vi "多IP测试.vi"() -> ()   [LabVIEW 2019]
uses:
  <vilib>/Utility/miscctls.llb/LVPointTypeDef.ctl
panel:
  out "本机IP":string
  out "16记录":string[][](table)
  out "06记录":string[][](table)
  out "03记录（去重）":string[][](table)
  in  "选项卡控件":T1(tab)
  in  "簇 1":T2 caption="寄存器模拟"
  in  "簇 2":T2 caption="寄存器模拟"
  in  "簇 3":T2 caption="寄存器模拟"
  in  "簇 4":T2 caption="寄存器模拟"
  in  "簇 5":T2 caption="寄存器模拟"
  in  "簇 6":T2 caption="寄存器模拟"
  in  "簇 7":T2 caption="寄存器模拟"
  in  "簇 8":T2 caption="寄存器模拟"
  in  "簇 9":T2 caption="寄存器模拟"
  in  "初始化数组":bool
  in  "复位":bool
  in  "停止":bool
  in  "服务端地址":string="127.0.0.1"
  in  "远程端口":u16=4001
  in  "本地设置":T3={"0"={"连接设置"=FALSE, "本地端口"=5001}, "1"={"连接设置"=FALSE, "本地端口"=5002}, "2"={"连接设置"=FALSE, "本地端口"=5003}, "3"={"连接设置"=FALSE, "本地端口"=5004}, "4"={"连接设置"=FALSE, "本地端口"=5005}, "5"={"连接设置"=FALSE, "本地端口"=5006}, "6"={"连接设置"=FALSE, "本地端口"=5007}, "7"={"连接设置"=FALSE, "本地端口"=5008}, "8"={"连接设置"=FALSE, "本地端口"=5009}}
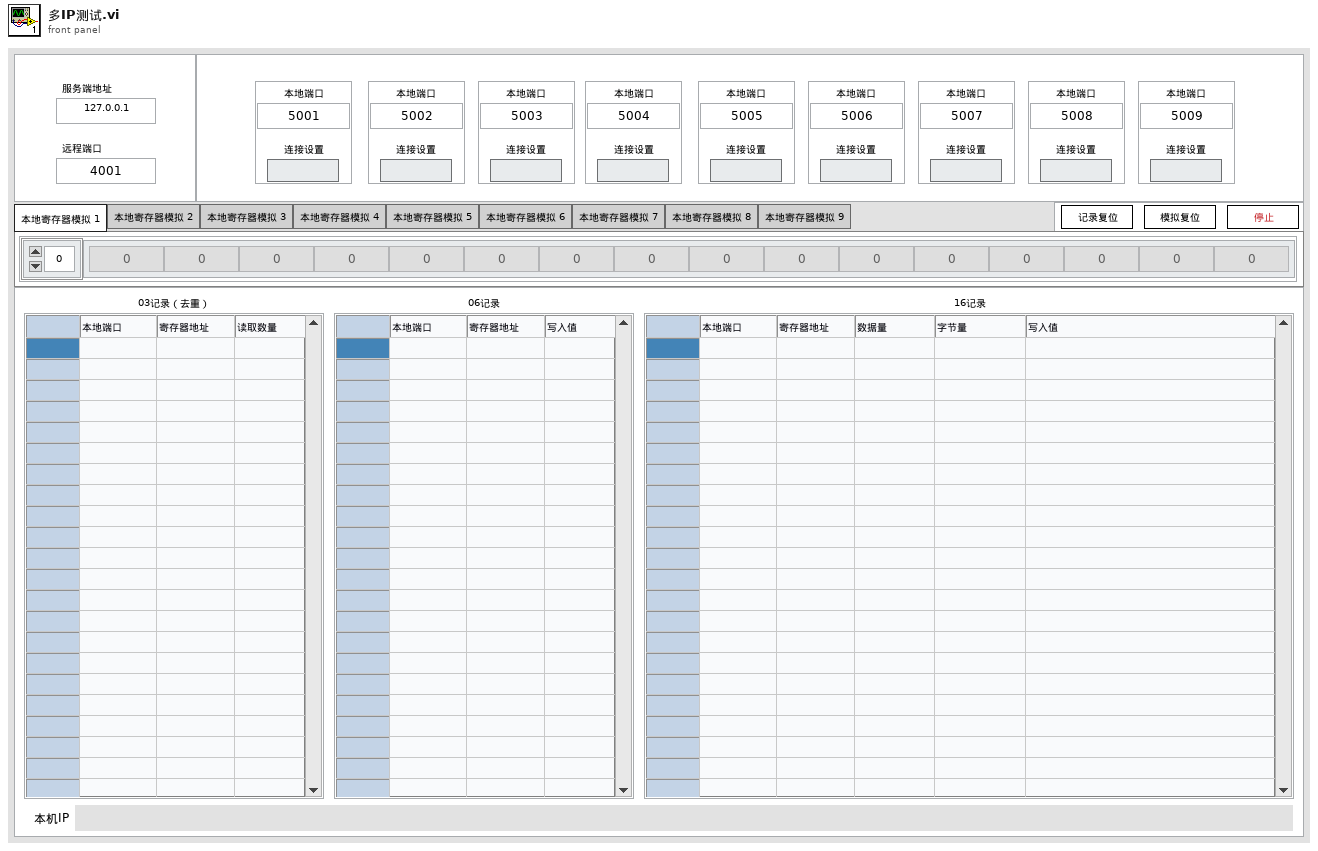
[diagram p1: front panel]
types:
  T1 = enum32{"本地寄存器模拟 1", "本地寄存器模拟 2", "本地寄存器模拟 3", "本地寄存器模拟 4", "本地寄存器模拟 5", "本地寄存器模拟 6", "本地寄存器模拟 7", "本地寄存器模拟 8", "本地寄存器模拟 9"}
  T2 = cluster{"03记录":string[][], "06记录":string[][], "16记录":string[][], "模拟数组":u16[]}
  T3 = cluster{"0":cluster{"连接设置":bool, "本地端口":u16}, "1":cluster{"连接设置":bool, "本地端口":u16}, "2":cluster{"连接设置":bool, "本地端口":u16}, "3":cluster{"连接设置":bool, "本地端口":u16}, "4":cluster{"连接设置":bool, "本地端口":u16}, "5":cluster{"连接设置":bool, "本地端口":u16}, "6":cluster{"连接设置":bool, "本地端口":u16}, "7":cluster{"连接设置":bool, "本地端口":u16}, "8":cluster{"连接设置":bool, "本地端口":u16}}
  T4 = typedef "LVPointTypeDef.ctl" = cluster{"Horizontal":i16, "Vertical":i16}
  T5 = cluster{"Label.Text":string, "NewVal":cluster{"连接设置":bool, "本地端口":u16}}
  T6 = cluster{"本地端口":u16, "模拟数组":u16[], "03记录":string[][], "06记录":string[][], "16记录":string[][]}
  T7 = cluster{"03记录":string[][], "06记录":string[][], "16记录":string[][], "模拟数组":u16[]}[]
  T8 = cluster{"本地端口":u16, u16[], "03记录":string[][], "06记录":string[][], "16记录":string[][]}
  T9 = cluster{"[0]":cluster{"连接设置":bool, "本地端口":u16}, "[1]":cluster{"连接设置":bool, "本地端口":u16}, "[2]":cluster{"连接设置":bool, "本地端口":u16}, "[3]":cluster{"连接设置":bool, "本地端口":u16}, "[4]":cluster{"连接设置":bool, "本地端口":u16}, "[5]":cluster{"连接设置":bool, "本地端口":u16}, "[6]":cluster{"连接设置":bool, "本地端口":u16}, "[7]":cluster{"连接设置":bool, "本地端口":u16}, "[8]":cluster{"连接设置":bool, "本地端口":u16}}
  T10 = cluster{"Value[0]":cluster{"连接设置":bool, "本地端口":u16}, "Value[1]":cluster{"连接设置":bool, "本地端口":u16}, "Value[2]":cluster{"连接设置":bool, "本地端口":u16}, "Value[3]":cluster{"连接设置":bool, "本地端口":u16}, "Value[4]":cluster{"连接设置":bool, "本地端口":u16}, "Value[5]":cluster{"连接设置":bool, "本地端口":u16}, "Value[6]":cluster{"连接设置":bool, "本地端口":u16}, "Value[7]":cluster{"连接设置":bool, "本地端口":u16}, "Value[8]":cluster{"连接设置":bool, "本地端口":u16}}
  T11 = cluster{"本地端口":u16, "模拟数组":u16[], "03记录":string[][], "06记录":string[][], "16记录":string[][]}[]
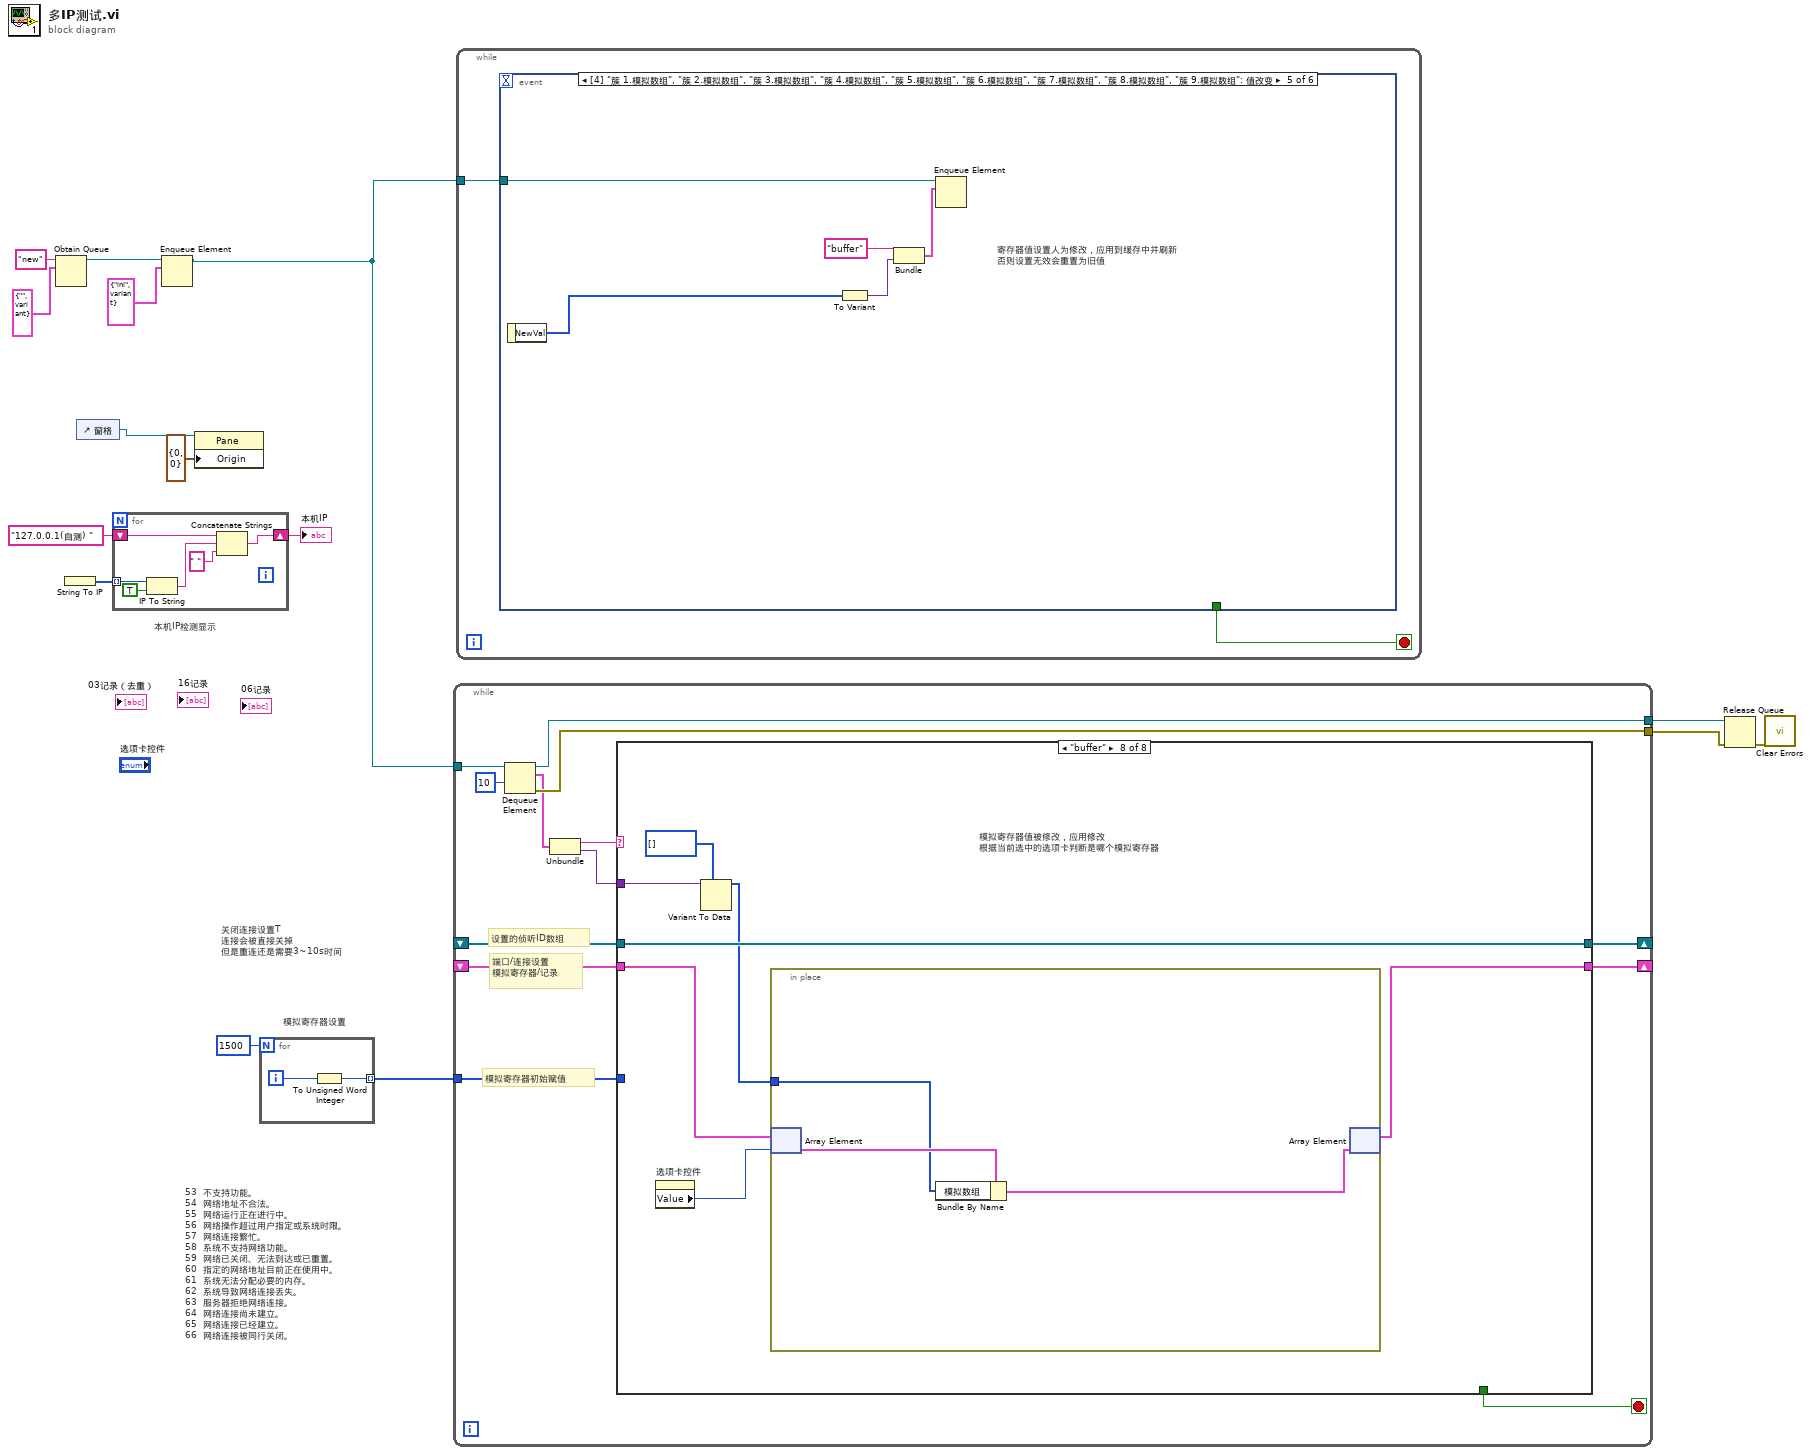
[diagram p0: block diagram]
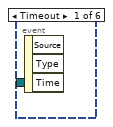
[diagram p2: hidden frame]
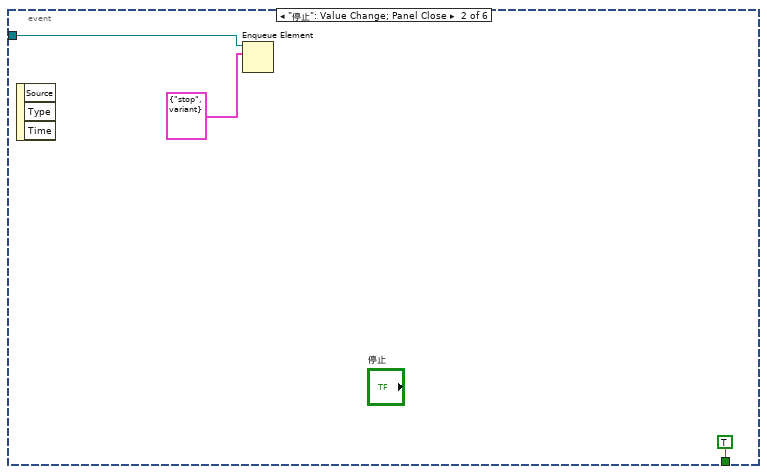
[diagram p3: hidden frame]
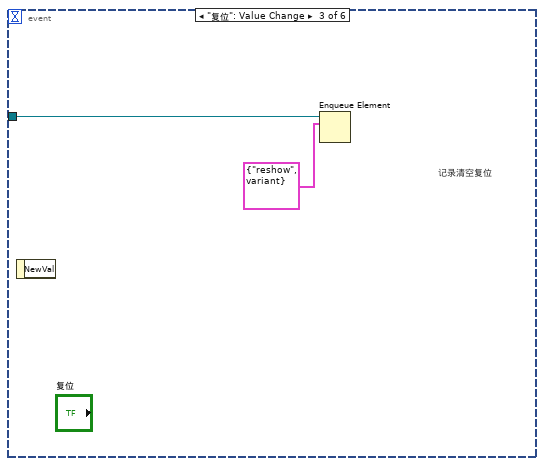
[diagram p4: hidden frame]
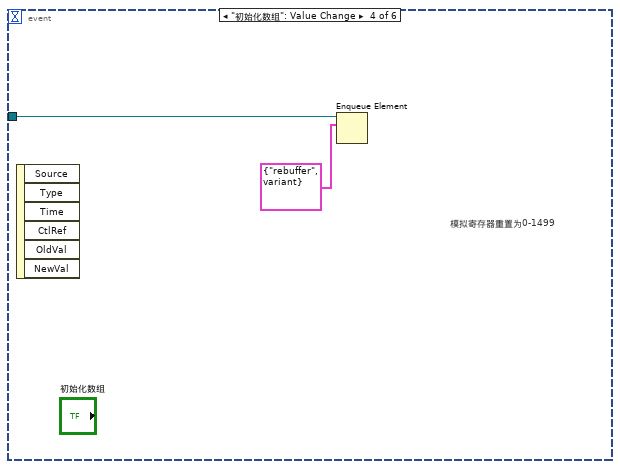
[diagram p5: hidden frame]
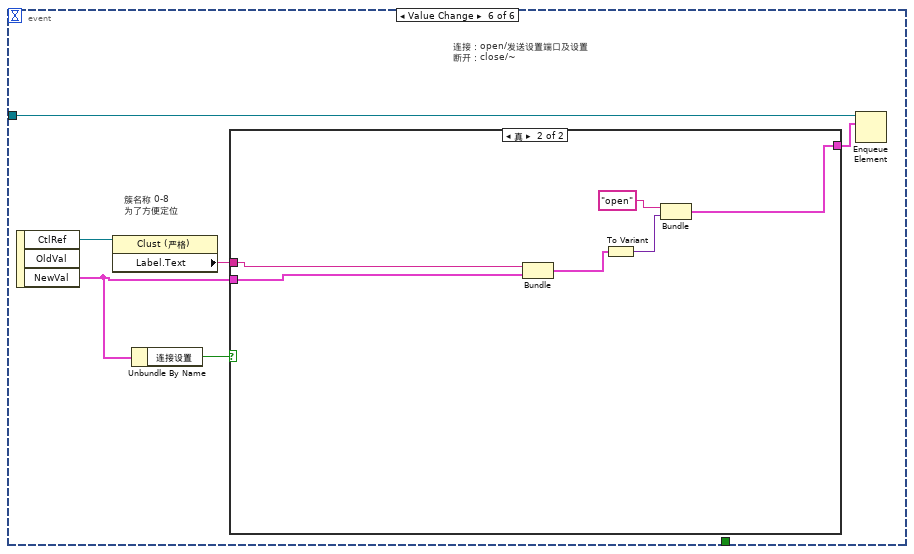
[diagram p6: hidden frame]
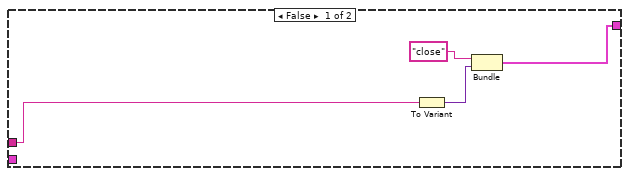
[diagram p7: hidden frame]
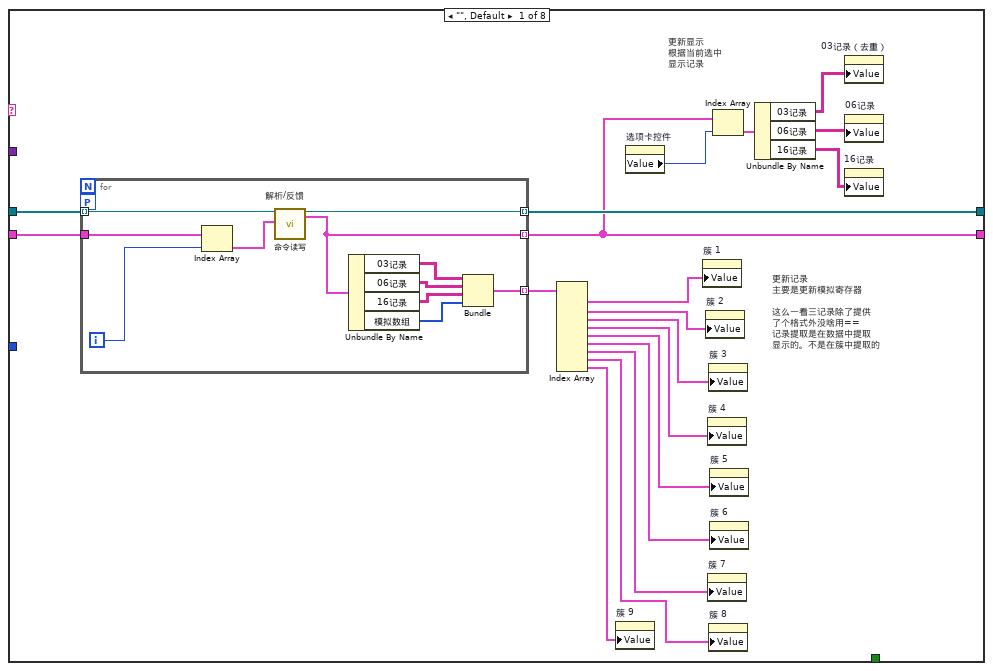
[diagram p8: hidden frame]
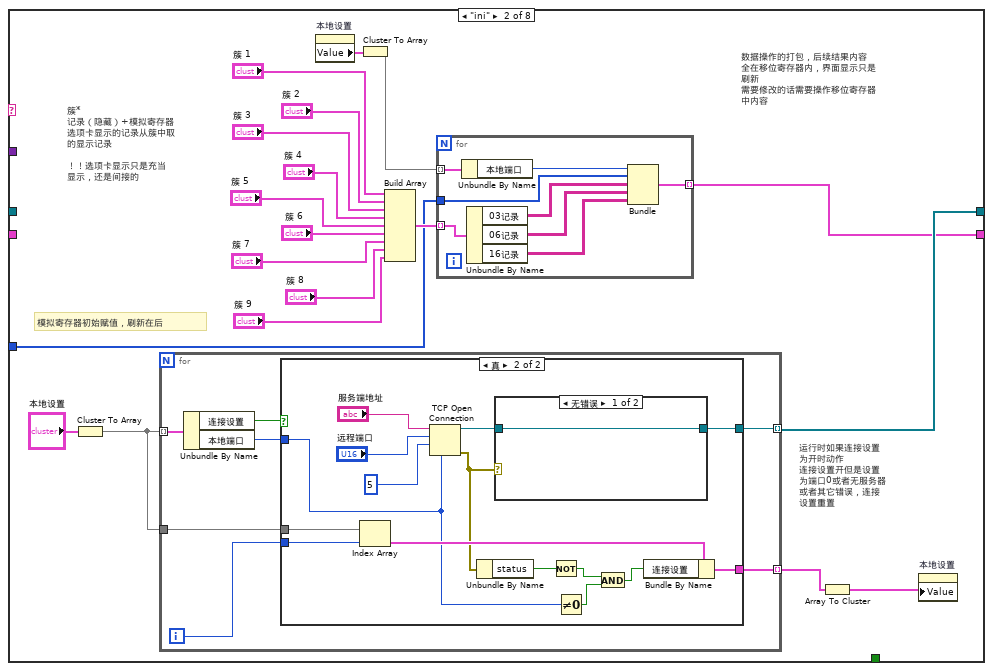
[diagram p9: hidden frame]
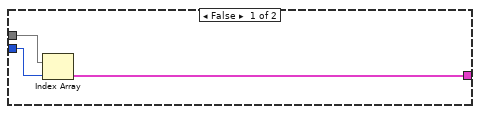
[diagram p10: hidden frame]
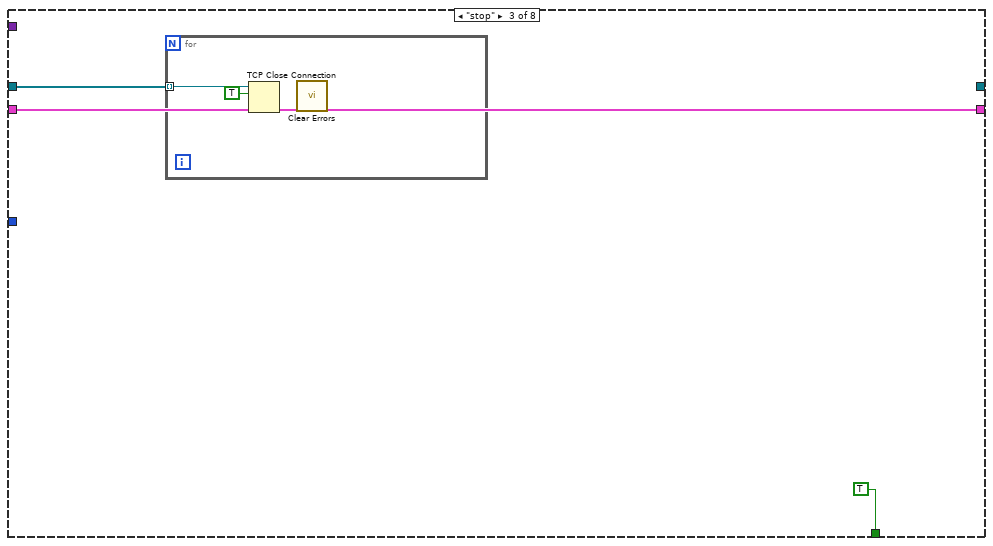
[diagram p12: hidden frame]
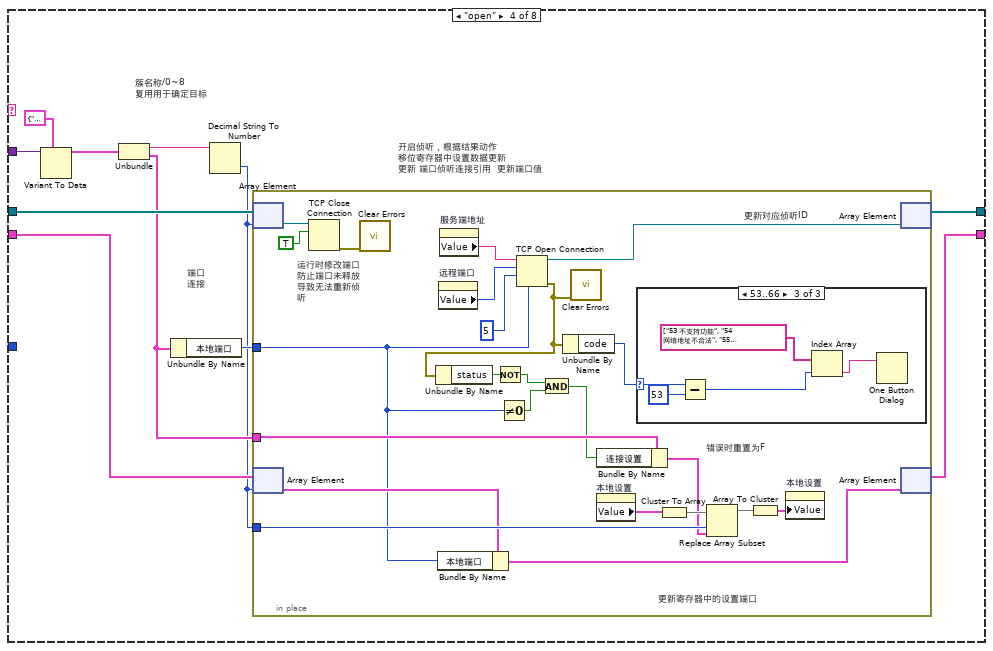
[diagram p13: hidden frame]
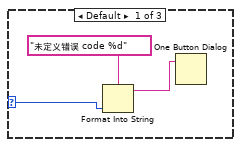
[diagram p14: hidden frame]
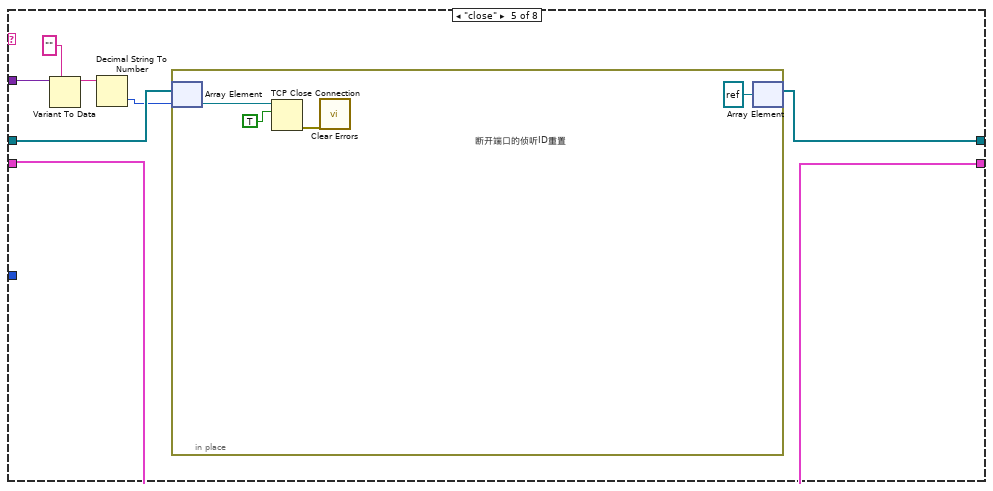
[diagram p16: hidden frame]
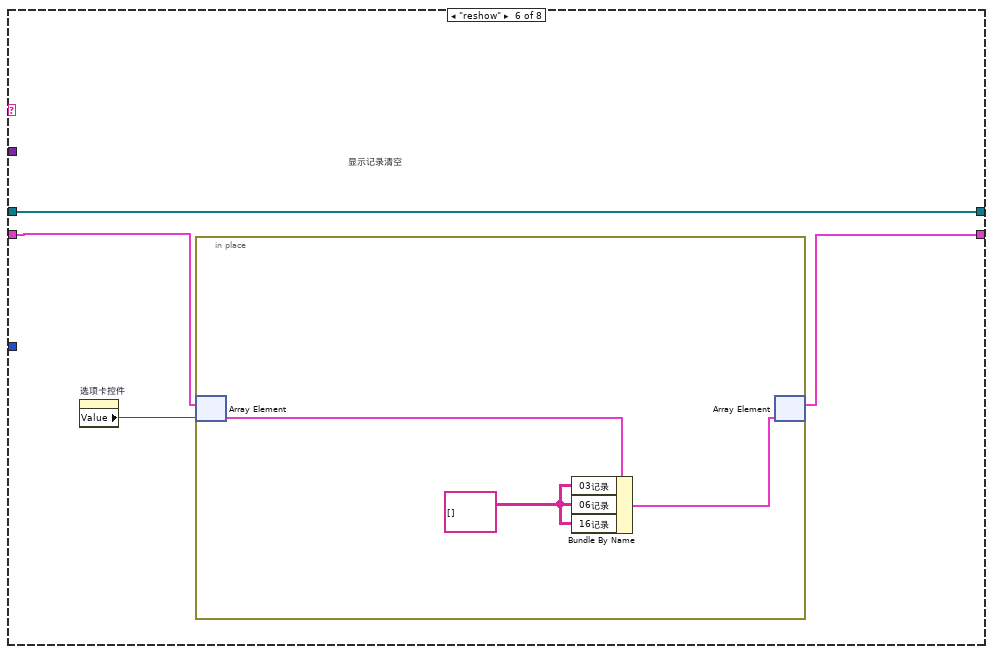
[diagram p17: hidden frame]
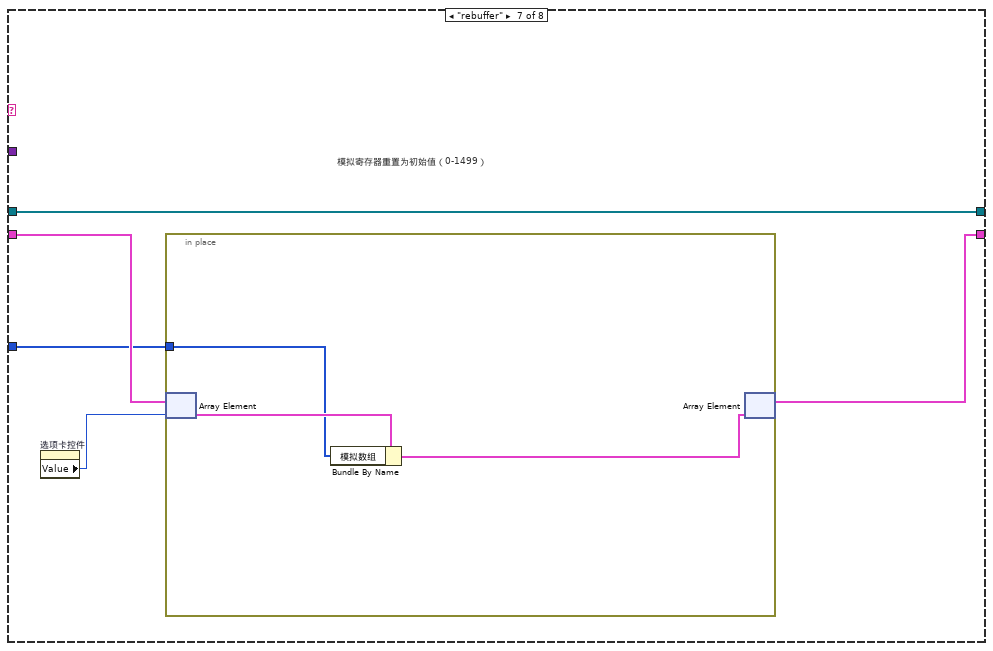
[diagram p18: hidden frame]
diagram:
  # "关闭连接设置T\n连接会被直接关掉\n但是重连还是需要3~10s时间"
  # "53  不支持功能。\n54  网络地址不合法。\n55  网络运行正在进行中。\n56  网络操作超过用户指定或系统时限。\n57  网络连接繁忙。\n58  系统不支持网络功能。\n59  网络已关闭、无法到达或已重置。\n60  指定的网络地址目前正在使用中。\n61  系统无法分配必要的内存。\n62  系统导致网络连接丢失。\n63  服务器拒绝网络连接。\n64  网络连接尚未建立。\n65  网络连接已经建立。\n66  网络连接被同行关闭。"
  # "本机IP检测显示"
  # "模拟寄存器设置"
  n1 = Obtain Queue(name (unnamed)="new" ("名称（未命名）"), element data type=cluster{"元素":string, variant} {"元素"="", variant}) -> (queue out=w14:refnum<queue>)  [unwired: 3 in, 2 out]
  n2 = String To IP() -> (0:w2:u32[])  [unwired: 1 in]
  n3 = control-ref of="窗格"() -> (w7:refnum<vi>)
  n4 = for {
    tunnel: w2 -> [w21] mode=indexing
    shift-right: [w18] -> w3
    shift-left: "127.0.0.1(自测) " ("name") -> [w19]
    n5 = IP To String(1:TRUE ("句点符号？(F)"), 2:w21) -> (0:w17:string)
    n6 = Concatenate Strings(w19, w17, " " ("字符串")) -> (w18:string)
  }
  "本机IP" <- w3
  n7 = Enqueue Element(queue=w14, element=cluster{"元素":string, variant} {"元素"="ini", variant}) -> (queue out=w8:refnum<queue>)  [unwired: 2 in, 2 out]
  n8 = property class="Pane"(reference=w7, "Origin"=T4 {"Horizontal"=0, "Vertical"=0} ("原点")) -> ()  [unwired: 1 in, 2 out]
  n9 = for {
    N: 1500 -> [_]
    tunnel: [w22] -> w4 mode=indexing
    i -> [w23]
    n10 = To Unsigned Word Integer(number=w23) -> (unsigned 16bit integer=w22:u16)
  }
  n11 = while {
    tunnel: w8 -> [w36]
    shift-right: [w35] -> _
    shift-left: _ -> [w30]
    tunnel: [w33] -> w12
    tunnel: [w32] -> w11
    shift-right: [w25] -> _
    shift-left: _ -> [w26]
    tunnel: w4 -> [w24]
    stop <- w34 stop-if-true
    # "设置的侦听ID数组"
    # "端口/连接设置\n模拟寄存器/记录"
    # "模拟寄存器初始赋值"
    n12 = Dequeue Element(queue=w36, timeout in ms (-1)=10 ("超时毫秒(-1)")) -> (queue out=w33:refnum<queue>, element=w29:cluster{"元素":string, variant}, error out=w32:errorcluster)  [unwired: 1 in, 1 out]
    n13 = Unbundle(w29) -> ("元素"=w28:string, w27:variant)
    n14 = case shown="\"buffer\"" w28 {
      tunnel: [w54 w84 _ w134 w172 w183 w191 w201] -> w35
      tunnel: [_ _ TRUE _ _ _ _ _] -> w34
      tunnel: w30 -> [w55 _ w121 w135 w171 w183 w191 w201]
      tunnel: w27 -> [_ _ _ w137 w174 _ _ w200]
      tunnel: w26 -> [w53 _ w122 w128 w169 w181 w189 w198]
      tunnel: [w52 w68 w122 w129 w169 w180 w188 w197] -> w25
      tunnel: w24 -> [_ w67 _ _ _ _ w187 _]
      frame "", Default {
        # "更新显示\n根据当前选中\n显示记录"
        # "更新记录\n主要是更新模拟寄存器\n\n这么一看三记录除了提供\n了个格式外没啥用==\n记录提取是在数据中提取\n显示的。不是在簇中提取的"
        n15 = for {
          tunnel: w55 -> [w66] mode=indexing
          tunnel: [w65] -> w54 mode=indexing
          tunnel: w53 -> [w63]
          tunnel: [w61] -> w52 mode=indexing
          tunnel: [w56] -> w46 mode=indexing
          workers-P: _ -> [_]
          i -> [w64]
          # "解析/反馈"
          n16 = Index Array(array=w63, index=w64) -> (element=w62:T6)
          n17 = call "命令读写.vi"("连接ID"=w66, "输入簇"=w62) -> ("连接ID输出"=w65:refnum<k5>, "输出簇"=w61:T6)  [unwired: 16 in]
          n18 = Unbundle By Name(w61) -> ("03记录"=w60:string[][], "06记录"=w59:string[][], "16记录"=w58:string[][], "模拟数组"=w57:u16[])
          n19 = Bundle("03记录"=w60, "06记录"=w59, "16记录"=w58, "模拟数组"=w57) -> (w56:T2)  [unwired: 1 in]
        }
        n20 = Index Array(array=w46) -> (element #1=w45:T2, element #2=w44:T2, element #3=w43:T2, element #4=w40:T2, element #5=w39:T2, element #6=w38:T2, element #7=w37:T2, element #8=w41:T2, element #9=w42:T2)  [unwired: 9 in]
        n21 = property on="簇 9" class="Clust (严格)"("Value"=w42) -> ()  [unwired: 2 in, 2 out]
        n22 = property on="选项卡控件" class="TabCtl (严格)"() -> ("Value"=w51:T1)  [unwired: 2 in, 2 out]
        n23 = property on="簇 1" class="Clust (严格)"("Value"=w45) -> ()  [unwired: 2 in, 2 out]
        n24 = property on="簇 2" class="Clust (严格)"("Value"=w44) -> ()  [unwired: 2 in, 2 out]
        n25 = property on="簇 4" class="Clust (严格)"("Value"=w40) -> ()  [unwired: 2 in, 2 out]
        n26 = property on="簇 7" class="Clust (严格)"("Value"=w37) -> ()  [unwired: 2 in, 2 out]
        n27 = property on="簇 3" class="Clust (严格)"("Value"=w43) -> ()  [unwired: 2 in, 2 out]
        n28 = property on="簇 8" class="Clust (严格)"("Value"=w41) -> ()  [unwired: 2 in, 2 out]
        n29 = property on="簇 5" class="Clust (严格)"("Value"=w39) -> ()  [unwired: 2 in, 2 out]
        n30 = property on="簇 6" class="Clust (严格)"("Value"=w38) -> ()  [unwired: 2 in, 2 out]
        n31 = Index Array(array=w52, index=w51) -> (element=w50:T6)
        n32 = Unbundle By Name(w50) -> ("03记录"=w47:string[][], "06记录"=w49:string[][], "16记录"=w48:string[][])
        n33 = property on="03记录（去重）" class="Tbl (严格)"("Value"=w47) -> ()  [unwired: 2 in, 2 out]
        n34 = property on="06记录" class="Tbl (严格)"("Value"=w49) -> ()  [unwired: 2 in, 2 out]
        n35 = property on="16记录" class="Tbl (严格)"("Value"=w48) -> ()  [unwired: 2 in, 2 out]
      }
      frame "ini" {
        # "数据操作的打包，后续结果内容\n全在移位寄存器内，界面显示只是\n刷新\n需要修改的话需要操作移位寄存器\n中内容"
        # "运行时如果连接设置\n为开时动作\n连接设置开但是设置\n为端口0或者无服务器\n或者其它错误，连接\n设置重置"
        # "模拟寄存器初始赋值，刷新在后"
        # "簇*\n记录（隐藏）+模拟寄存器\n选项卡显示的记录从簇中取\n的显示记录\n\n！！选项卡显示只是充当\n显示，还是间接的"
        n36 = Cluster To Array(cluster="本地设置") -> (array=w83:cluster{"连接设置":bool, "本地端口":u16}[])
        n37 = for {
          tunnel: w83 -> [w100] mode=indexing
          tunnel: [w97] -> w84 mode=indexing
          tunnel: w83 -> [w96]
          tunnel: [w94] -> w81 mode=indexing
          i -> [w95]
          n38 = Unbundle By Name(w100) -> ("连接设置"=w99:bool, "本地端口"=w98:u16)
          n39 = case shown="真" w99 {
            tunnel: w98 -> [_ w107]
            tunnel: [_ w115] -> w97
            tunnel: w96 -> [w102 w113]
            tunnel: w95 -> [w103 w112]
            tunnel: [w101 w109] -> w94
            frame False {
              n40 = Index Array(array=w102, index=w103) -> (element=w101:cluster{"连接设置":bool, "本地端口":u16})
            }
            frame True {
              n41 = Index Array(array=w113, index=w112) -> (element=w111:cluster{"连接设置":bool, "本地端口":u16})
              n42 = TCP Open Connection(address="服务端地址", remote port or service name="远程端口", timeout ms (60000)=5 ("超时毫秒(60000)"), local port=w107) -> (connection ID=w114:refnum<k5>, error out=w110:errorcluster)  [unwired: 1 in]
              n43 = Unbundle By Name(w110) -> ("status"=w108:bool)
              n44 = case shown="无错误" w110 {
                tunnel: [w119 w120] -> w115
                tunnel: w114 -> [w119 w120]
                frame No Error {
                }
                frame Default {
                }
              }
              n45 = Not(x=w108) -> (.not. x?=w106:bool)
              n46 = Not Equal To 0?(x=w107) -> (x != 0?=w105:bool)
              n47 = And(x=w106, y=w105) -> (x .and. y?=w104:bool)
              n48 = Bundle By Name(cluster=w111, "连接设置"=w104) -> (w109:cluster{"连接设置":bool, "本地端口":u16})
            }
          }
        }
        n49 = property on="本地设置" class="Clust (严格)"() -> ("Value"=w78:T3)  [unwired: 2 in, 2 out]
        n50 = Cluster To Array(cluster=w78) -> (array=w79:cluster{"连接设置":bool, "本地端口":u16}[])
        n51 = Build Array("簇 1", "簇 2", "簇 3", "簇 4", "簇 5", "簇 6", "簇 7", "簇 8", "簇 9") -> (w80:T7)
        n52 = for {
          tunnel: w79 -> [w93] mode=indexing
          tunnel: w80 -> [w90] mode=indexing
          tunnel: [w92] -> w68 mode=indexing
          tunnel: w67 -> [w86]
          n53 = Unbundle By Name(w93) -> ("本地端口"=w91:u16)
          n54 = Unbundle By Name(w90) -> ("03记录"=w89:string[][], "06记录"=w88:string[][], "16记录"=w87:string[][])
          n55 = Bundle("本地端口"=w91, w86, "03记录"=w89, "06记录"=w88, "16记录"=w87) -> (w92:T8)  [unwired: 1 in]
        }
        n56 = Array To Cluster(array=w81) -> (cluster=w82:T9)
        n57 = property on="本地设置" class="Clust (严格)"("Value"=w82) -> ()  [unwired: 2 in, 2 out]
      }
      frame "stop" {
        n58 = for {
          tunnel: w121 -> [w125] mode=indexing
          n59 = TCP Close Connection(connection ID=w125, abort (F)=TRUE ("中止(F)")) -> (error out=w126:errorcluster)  [unwired: 1 in, 1 out]
          n60 = call <vilib>:"Clear Errors.vi"("error in (no error)"=w126) -> ()  [unwired: 5 in, 2 out]
        }
      }
      frame "open" {
        # "端口\n连接"
        # "簇名称/0~8\n复用用于确定目标"
        # "开启侦听，根据结果动作\n移位寄存器中设置数据更新\n更新 端口侦听连接引用  更新端口值"
        n61 = Variant To Data(type=T5 {"Label.Text"="", "NewVal"={"连接设置"=FALSE, "本地端口"=0}} ("输出簇"), Variant=w137) -> (data=w136:T5)  [unwired: 1 in, 1 out]
        n62 = Unbundle(w136) -> ("Label.Text"=w131:string, "NewVal"=w130:cluster{"连接设置":bool, "本地端口":u16})
        n63 = Unbundle By Name(w130) -> ("本地端口"=w133:u16)
        n64 = Decimal String To Number(string=w131) -> (number=w127:i32)  [unwired: 2 in, 1 out]
        n65 = in-place {
          in-place-border: w133 -> [w144]
          in-place-border: w127 -> [w151]
          in-place-border: w130 -> [w150]
          # "运行时修改端口\n防止端口未释放\n导致无法重新侦\n听"
          # "更新寄存器中的设置端口"
          # "更新对应侦听ID"
          # "错误时重置为F"
          n66 = in-place-array #1(w135, w127) -> (w142:refnum<k5>)
          n67 = in-place-array #2(w128, w127) -> (w145:T6)
          n68 = TCP Close Connection(connection ID=w142, abort (F)=TRUE ("中止(F)")) -> (error out=w141:errorcluster)  [unwired: 1 in, 1 out]
          n69 = call <vilib>:"Clear Errors.vi"("error in (no error)"=w141) -> ()  [unwired: 5 in, 2 out]
          n70 = Bundle By Name(cluster=w145, "本地端口"=w144) -> (w143:T6)
          n71 = property on="远程端口" class="DigNum (严格)"() -> ("Value"=w158:u16)  [unwired: 2 in, 2 out]
          n72 = property on="服务端地址" class="Str"() -> ("Value"=w159:string)  [unwired: 2 in, 2 out]
          n73 = Not Equal To 0?(x=w144) -> (x != 0?=w156:bool)
          n74 = TCP Open Connection(address=w159, remote port or service name=w158, timeout ms (60000)=5 ("超时毫秒(60000)"), local port=w144) -> (connection ID=w157:refnum<k5>, error out=w140:errorcluster)  [unwired: 1 in]
          n75 = Unbundle By Name(w140) -> ("status"=w154:bool)
          n76 = Not(x=w154) -> (.not. x?=w155:bool)
          n77 = And(x=w155, y=w156) -> (x .and. y?=w146:bool)
          n78 = Unbundle By Name(w140) -> ("code"=w139:i32)
          n79 = call <vilib>:"Clear Errors.vi"("error in (no error)"=w140) -> ()  [unwired: 5 in, 2 out]
          n80 = Bundle By Name(cluster=w150, "连接设置"=w146) -> (w149:cluster{"连接设置":bool, "本地端口":u16})
          n81 = property on="本地设置" class="Clust (严格)"() -> ("Value"=w152:T3)  [unwired: 2 in, 2 out]
          n82 = case shown="53..66" w139 {
            selector: w139 -> [w163 _ w168]
            frame Default {
              n83 = Format Into String(format string="未定义错误 code %d" ("格式字符串"), w163) -> (resulting string=w162:string)  [unwired: 2 in, 1 out]
              n84 = One Button Dialog(message=w162) -> ()  [unwired: 1 in, 1 out]
            }
            frame 0 {
            }
            frame 53..66 {
              n85 = Subtract(x=w168, y=53) -> (x-y=w165:i32)
              n86 = Index Array(array=string[] ["53 不支持功能", "54 网络地址不合法", "55 网络运行正在进行中", "56 网络操作超过用户指定或系统时限", "57 网络连接繁忙", "58 系统不支持网络功能", "59 网络已关闭、无法到达或已重置。", "60 指定的网络地址目前正在使用中", "61 系统无法分配必要的内存", "62 系统导致网络连接丢失", "63 服务器拒绝网络连接", "64 网络连接尚未建立", "65 网络连接已经建立", "66 网络连接被同行关闭"], index=w165) -> (element=w164:string)
              n87 = One Button Dialog(message=w164) -> ()  [unwired: 1 in, 1 out]
            }
          }
          n88 = Cluster To Array(cluster=w152) -> (array=w153:cluster{"连接设置":bool, "本地端口":u16}[])
          n89 = Replace Array Subset(array=w153, new element=w149, index=w151) -> (w148:cluster{"连接设置":bool, "本地端口":u16}[])
          n90 = Array To Cluster(array=w148) -> (cluster=w147:T10)
          n91 = property on="本地设置" class="Clust (严格)"("Value"=w147) -> ()  [unwired: 2 in, 2 out]
          n92 = in-place-array #1(w157) -> (w134:refnum<k5>[])  [unwired: 1 out]
          n93 = in-place-array #2(w143) -> (w129:T11)  [unwired: 1 out]
        }
      }
      frame "close" {
        n94 = Variant To Data(type="", Variant=w174) -> (data=w173:string)  [unwired: 1 in, 1 out]
        n95 = Decimal String To Number(string=w173) -> (number=w170:i32)  [unwired: 2 in, 1 out]
        n96 = in-place {
          # "断开端口的侦听ID重置"
          n97 = in-place-array #3(w171, w170) -> (w178:refnum<k5>)
          n98 = TCP Close Connection(connection ID=w178, abort (F)=TRUE ("中止(F)")) -> (error out=w177:errorcluster)  [unwired: 1 in, 1 out]
          n99 = call <vilib>:"Clear Errors.vi"("error in (no error)"=w177) -> ()  [unwired: 5 in, 2 out]
          n100 = in-place-array #3(refnum<k5> refnum ("元素")) -> (w172:refnum<k5>[])  [unwired: 1 out]
        }
      }
      frame "reshow" {
        # "显示记录清空"
        n101 = property on="选项卡控件" class="TabCtl (严格)"() -> ("Value"=w182:T1)  [unwired: 2 in, 2 out]
        n102 = in-place {
          w185 = string[][] [] ("03记录")
          n103 = in-place-array #4(w181, w182) -> (w184:T6)
          n104 = Bundle By Name(cluster=w184, "03记录"=w185, "06记录"=w185, "16记录"=w185) -> (w186:T6)
          n105 = in-place-array #4(w186) -> (w180:T11)  [unwired: 1 out]
        }
      }
      frame "rebuffer" {
        # "模拟寄存器重置为初始值（0-1499）"
        n106 = property on="选项卡控件" class="TabCtl (严格)"() -> ("Value"=w190:T1)  [unwired: 2 in, 2 out]
        n107 = in-place {
          in-place-border: w187 -> [w193]
          n108 = in-place-array #5(w189, w190) -> (w194:T6)
          n109 = Bundle By Name(cluster=w194, "模拟数组"=w193) -> (w192:T6)
          n110 = in-place-array #5(w192) -> (w188:T11)  [unwired: 1 out]
        }
      }
      frame "buffer" {
        # "模拟寄存器值被修改，应用修改\n根据当前选中的选项卡判断是哪个模拟寄存器"
        n111 = property on="选项卡控件" class="TabCtl (严格)"() -> ("Value"=w195:T1)  [unwired: 2 in, 2 out]
        n112 = Variant To Data(type=u16[] [] ("新值"), Variant=w200) -> (data=w196:u16[])  [unwired: 1 in, 1 out]
        n113 = in-place {
          in-place-border: w196 -> [w203]
          n114 = in-place-array #6(w198, w195) -> (w204:T6)
          n115 = Bundle By Name(cluster=w204, "模拟数组"=w203) -> (w202:T6)
          n116 = in-place-array #6(w202) -> (w197:T11)  [unwired: 1 out]
        }
      }
    }
  }
  n117 = while {
    tunnel: w8 -> [w206]
    stop <- w205 stop-if-true
    n118 = event shown="[4] \"簇 1.模拟数组\", \"簇 2.模拟数组\", \"簇 3.模拟数组\", \"簇 4.模拟数组\", \"簇 5.模拟数组\", \"簇 6.模拟数组\", \"簇 7.模拟数组\", \"簇 8.模拟数组\", \"簇 9.模拟数组\": 值改变" {
      selector: _ -> [_ _ _ _ _ _]
      dyn-events: _ -> [_ _ _ _ _ _]
      timeout: _ -> [_ _ _ _ _ _]
      tunnel: w206 -> [_ w209 w210 w212 w214 w224]
      tunnel: [_ TRUE ("停止") _ _ _ _] -> w205
      event Timeout {
        n119 = event-data() -> ()  [unwired: 1 in, 3 out]
      }
      event "停止": Value Change; Panel Close {
        n120 = event-data() -> ()  [unwired: 1 in, 3 out]
        n121 = Enqueue Element(queue=w209, element=cluster{"元素":string, variant} {"元素"="stop", variant}) -> ()  [unwired: 2 in, 3 out]
      }
      event "复位": Value Change {
        # "记录清空复位"
        n122 = event-data() -> ()  [unwired: 1 in, 1 out]
        n123 = Enqueue Element(queue=w210, element=cluster{"元素":string, variant} {"元素"="reshow", variant}) -> ()  [unwired: 2 in, 3 out]
      }
      event "初始化数组": Value Change {
        # "模拟寄存器重置为0-1499"
        n124 = event-data() -> ()  [unwired: 1 in, 6 out]
        n125 = Enqueue Element(queue=w212, element=cluster{"元素":string, variant} {"元素"="rebuffer", variant}) -> ()  [unwired: 2 in, 3 out]
      }
      event "簇 1.模拟数组", "簇 2.模拟数组", "簇 3.模拟数组", "簇 4.模拟数组", "簇 5.模拟数组", "簇 6.模拟数组", "簇 7.模拟数组", "簇 8.模拟数组", "簇 9.模拟数组": Value Change {
        # "寄存器值设置人为修改，应用到缓存中并刷新\n否则设置无效会重置为旧值"
        n126 = event-data() -> ("NewVal"=w218:u16[])  [unwired: 1 in]
        n127 = To Variant(anything=w218) -> (Variant=w216:variant)
        n128 = Bundle("元素"="buffer", "Variant"=w216) -> (w215:cluster{"元素":string, "Variant":variant})  [unwired: 1 in]
        n129 = Enqueue Element(queue=w214, element=w215) -> ()  [unwired: 2 in, 3 out]
      }
      event "本地设置.0", "本地设置.1", "本地设置.2", "本地设置.3", "本地设置.4", "本地设置.5", "本地设置.6", "本地设置.7", "本地设置.8": Value Change {
        # "簇名称 0-8\n为了方便定位"
        # "连接：open/发送设置端口及设置\n断开：close/~"
        n130 = event-data() -> ("CtlRef"=w222:refnum<vi>, "NewVal"=w219:cluster{"连接设置":bool, "本地端口":u16})  [unwired: 1 in, 1 out]
        n131 = property class="Clust (严格)"(reference=w222) -> ("Label.Text"=w221:string)  [unwired: 1 in, 2 out]
        n132 = Unbundle By Name(w219) -> ("连接设置"=w223:bool)
        n133 = case shown="真" w223 {
          tunnel: w221 -> [w225 w233]
          tunnel: [w226 w234] -> w220
          tunnel: w219 -> [_ w232]
          frame False {
            n134 = To Variant(anything=w225) -> (Variant=w228:variant)
            n135 = Bundle("元素"="close", "Variant"=w228) -> (w226:cluster{"元素":string, "Variant":variant})  [unwired: 1 in]
          }
          frame True {
            n136 = Bundle("Label.Text"=w233, "NewVal"=w232) -> (w229:T5)  [unwired: 1 in]
            n137 = To Variant(anything=w229) -> (Variant=w231:variant)
            n138 = Bundle("元素"="open", "Variant"=w231) -> (w234:cluster{"元素":string, "Variant":variant})  [unwired: 1 in]
          }
        }
        n139 = Enqueue Element(queue=w224, element=w220) -> ()  [unwired: 2 in, 3 out]
      }
    }
  }
  n140 = Release Queue(queue=w12, error in (no error)=w11) -> (error out=w13:errorcluster)  [unwired: 1 in, 2 out]
  n141 = call <vilib>:"Clear Errors.vi"("error in (no error)"=w13) -> ()  [unwired: 5 in, 2 out]
